vi "oa_Check Reset (N Channels).vi"(7 "reset?":bool=TRUE, 8 "error in (no error)":errorcluster, 10 "empty?":bool, 11 "resampled signal":cluster{"r0":dbl, "dr":dbl, "Y":dbl[]}[](array[cluster]) {"r0" format="%.2p"; "dr" format="%.2p"; "Y" format="%.2f"}) -> (0 "error out":errorcluster, 2 "reset?":bool, 3 "resampled signal out":cluster{"r0":dbl, "dr":dbl, "Y":dbl[]}[](array[cluster]))   [LabVIEW 2017, in "SoundVib_Resampling.lvlib"]
uses:
  <vilib>/addons/Sound and Vibration/Order Analysis/Resample Order Tracking/SoundVib_Resampling.lvlib
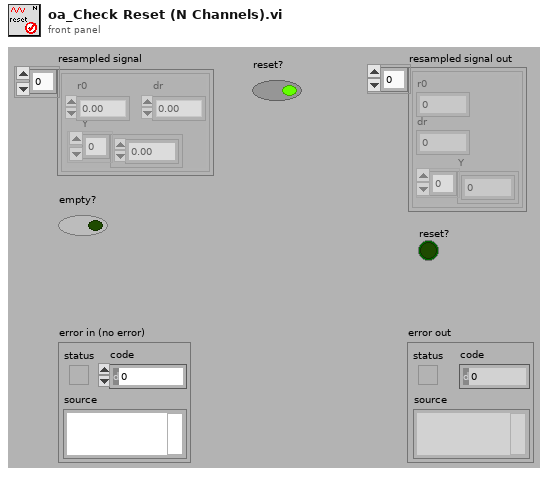
[diagram p1: front panel]
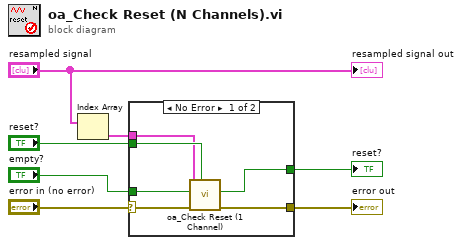
[diagram p0: block diagram]
diagram:
  n1 = Index Array(array="resampled signal") -> (element=w1:cluster{"r0":dbl, "dr":dbl, "Y":dbl[]})  [unwired: 1 in]
  n2 = case shown="No Error" "error in (no error)" {
    selector: "error in (no error)" -> [w13 w14]
    tunnel: [w12 w14] -> w6
    tunnel: "empty?" -> [w11 _]
    tunnel: "reset?" -> [w10 w15]
    tunnel: [w9 w15] -> w3
    tunnel: w1 -> [w8 _]
    frame No Error {
      n3 = call <vilib>:"oa_Check Reset (1 Channel).vi"("reset?"=w10, "error in (no error)"=w13, "empty signal?"=w11, "resampled signal"=w8) -> ("error out"=w12:errorcluster, "reset out?"=w9:bool)  [unwired: 5 in, 1 out]
    }
    frame Error {
    }
  }
  "error out" <- w6
  "reset?" <- w3
  "resampled signal out" <- "resampled signal"
